vi "Get Target Type.vi"(8 "error in":errorcluster, 11 "item in":T2 format="%.0x") -> (0 "error out":errorcluster, 2 "target type":T1=enum."Windows", 3 "item out":T2 format="%.0x")   [LabVIEW 2027, in "Embedded Data Logger Scripting.lvlib"]
uses:
  Embedded Data Logger Scripting.lvlib
  C:/NetCore/niveristand-embedded-data-logger-custom-device/Source/Scripting/Utility/Get Target Type.vi/NationalInstruments.VeriStand.SystemDefinitionAPI
  NationalInstruments.VeriStand.SystemDefinitionAPI
  <vilib>/NI VeriStand/Custom Device API/Custom Device Target Type.ctl
  <vilib>/NI VeriStand/Custom Device API/Custom Device API.lvlib
  C:/NetCoreDLL/NationalInstruments.VeriStand.SystemDefinitionAPI.dll
  NetCoreDLL/NationalInstruments.VeriStand.SystemDefinitionAPI.dll
  <vilib>/NI VeriStand/Custom Device API/Custom Device Item Ref.ctl
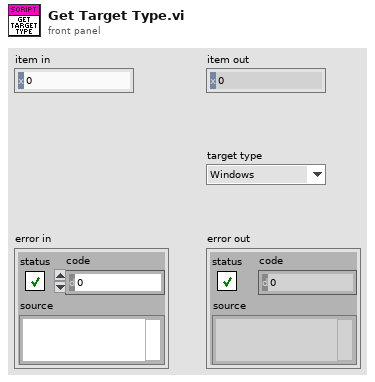
[diagram p1: front panel]
types:
  T1 = typedef "Custom Device API.lvlib/Custom Device Target Type.ctl" = enum16{"PharLap", "VxWorks", "Windows", "Linux_32_ARM", "Linux_x64"}
  T2 = typedef "Custom Device API.lvlib/Custom Device Item Ref.ctl" = u64
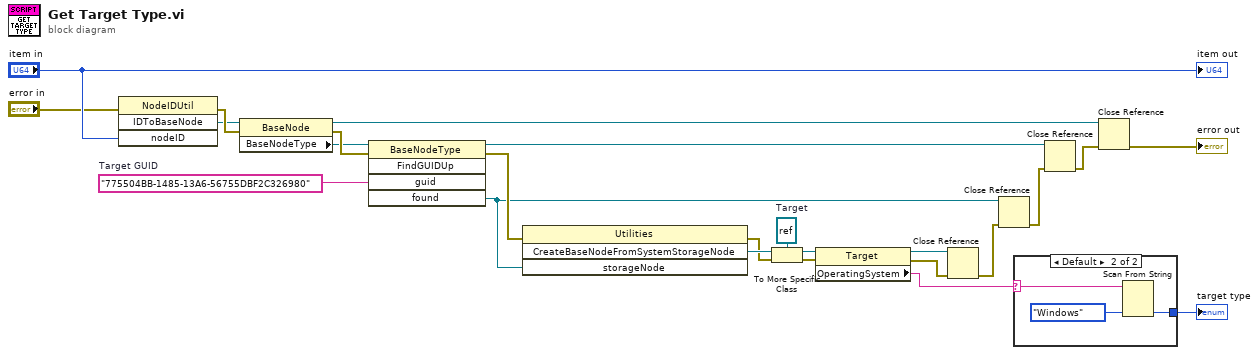
[diagram p0: block diagram]
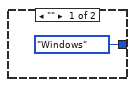
[diagram p2: hidden frame]
diagram:
  w21 = refnum<k39> refnum  # Target
  w24 = "775504BB-1485-13A6-56755DBF2C326980"  # Target GUID
  n1 = invoke class="NodeIDUtil" method="IDToBaseNode"(error in="error in", "nodeID"="item in") -> (error out=w18:errorcluster, "IDToBaseNode"=w6:refnum<k39>)  [unwired: 2 in, 2 out]
  n2 = property class="BaseNode"(reference=w6, error in=w18) -> (reference out=w10:refnum<k39>, error out=w17:errorcluster, "BaseNodeType"=w7:refnum<k39>)
  n3 = invoke class="BaseNodeType" method="FindGUIDUp"(reference=w7, error in=w17, "guid"=w24) -> (reference out=w12:refnum<k39>, error out=w5:errorcluster, "found"=w4:refnum<k39>)  [unwired: 2 in, 2 out]
  n4 = invoke class="Utilities" method="CreateBaseNodeFromSystemStorageNode"(error in=w5, "storageNode"=w4) -> (error out=w19:errorcluster, "CreateBaseNodeFromSystemStorageNode"=w22:refnum<k39>)  [unwired: 2 in, 2 out]
  n5 = To More Specific Class(target class=w21, reference=w22, error in=w19) -> (specific class reference=w20:refnum<k39>, error out=w16:errorcluster)
  n6 = property class="Target"(reference=w20, error in=w16) -> (reference out=w14:refnum<k39>, error out=w15:errorcluster, "OperatingSystem"=w2:string)
  n7 = Close Reference(reference=w14, error in (no error)=w15) -> (error out=w13:errorcluster)
  n8 = Close Reference(reference=w4, error in (no error)=w13) -> (error out=w11:errorcluster)
  n9 = case shown="Default" w2 {
    selector: w2 -> [_ w27]
    tunnel: [Custom_Device_Target_Type."Windows" ("Target Type") w26] -> w1
    frame "" {
    }
    frame Default {
      n10 = Scan From String(input string=w27, default 1=Custom_Device_Target_Type."Windows" ("Target Type")) -> (output 1=w26:T1)  [unwired: 3 in, 3 out]
    }
  }
  "target type" <- w1
  n11 = Close Reference(reference=w12, error in (no error)=w11) -> (error out=w9:errorcluster)
  n12 = Close Reference(reference=w10, error in (no error)=w9) -> (error out=→"error out":errorcluster)
  "item out" <- "item in"
